vi "half (x + y) [DBL].vi"(4 "y":dbl, 5 "x":dbl) -> (1 "(x+y)/2":dbl)   [LabVIEW 2019]
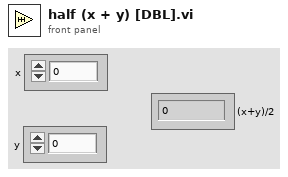
[diagram p1: front panel]
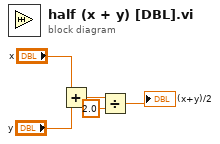
[diagram p0: block diagram]
diagram:
  n1 = Add(x="x", y="y") -> (x+y=w2:dbl)
  n2 = Divide(x=w2, y=2.0) -> (x/y=→"(x+y)/2":dbl)
